vi "rt_auto_disp.vi"(2 "Mean":dbl=1.0, 3 "Enable":bool) -> (1 "Dispense":bool)   [LabVIEW 2013]
uses:
  <vilib>/gmath/statdist.llb/Poisson Random.vi
  <vilib>/gmath/NI_Gmath.lvlib
panel:
  out "Timer value when Poisson\n number was generated":u32
  out "Poisson":u32
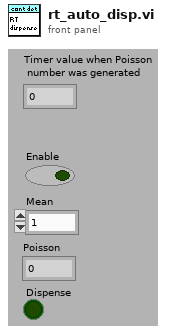
[diagram p1: front panel]
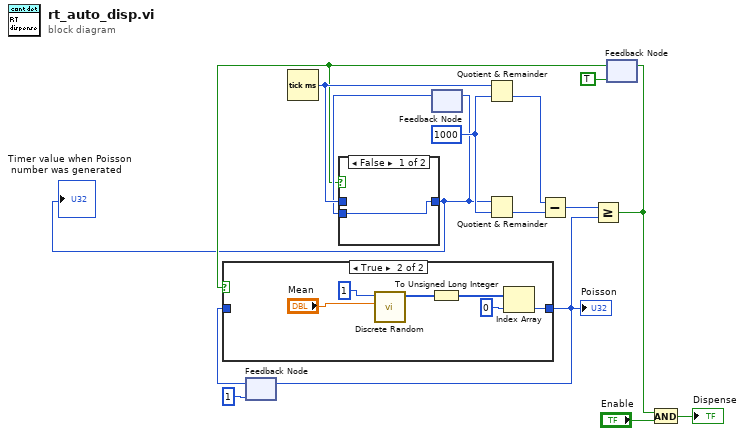
[diagram p0: block diagram]
diagram:
  w6 = u32 1000 ("y")
  n1 = feedback #1(u32 1 ("Numeric")) -> (w5:u32)
  n2 = Tick Count (ms)() -> (millisecond timer value=w15:u32)
  n3 = feedback #2() -> (w11:u32)  [unwired: 1 in]
  n4 = Quotient & Remainder(x=w15, y=w6) -> (floor(x/y)=w13:u32)  [unwired: 1 out]
  n5 = feedback #3(TRUE) -> (w9:bool)
  n6 = case shown="True" w9 {
    tunnel: [w16 w17] -> w8
    tunnel: w5 -> [w16 _]
    frame False {
    }
    frame True {
      n7 = call-poly <vilib>:"Discrete Random.vi"("lambda"="Mean", "samples"=1) -> ("Poisson random data"=w19:i32[])  [unwired: 8 in, 1 out]
      n8 = To Unsigned Long Integer(number=w19) -> (unsigned 32bit integer=w18:u32[])
      n9 = Index Array(array=w18, index=0) -> (element=w17:u32)
    }
  }
  "Poisson" <- w8
  n10 = feedback-in #1(w8) -> ()
  n11 = case shown="False" w9 {
    tunnel: [w23 w24] -> w1
    tunnel: w15 -> [_ w24]
    tunnel: w11 -> [w23 _]
    frame False {
    }
    frame True {
    }
  }
  "Timer value when Poisson\n number was generated" <- w1
  n12 = feedback-in #2(w1) -> ()
  n13 = Quotient & Remainder(x=w1, y=w6) -> (floor(x/y)=w7:u32)  [unwired: 1 out]
  n14 = Subtract(x=w13, y=w7) -> (x-y=w14:u32)
  n15 = Greater Or Equal?(x=w14, y=w8) -> (x >= y?=w10:bool)
  n16 = feedback-in #3(w10) -> ()
  n17 = And(x=w10, y="Enable") -> (x .and. y?=→"Dispense":bool)
